vi "Listener.vi"(8 "ErrorArray":errorcluster[](array[cluster])) -> (0 "ErrorArray":errorcluster[](array[cluster]), 2 "Accepted?":bool)   [LabVIEW 2017, in "Comms.lvlib"]
uses:
  Comms.lvlib
  <userlib>/NIST/Socket Class/Classes/Socket.TCP/Socket.TCP.lvclass
  <userlib>/NIST/NISTErrorLib/NISTErrorLib.lvlib
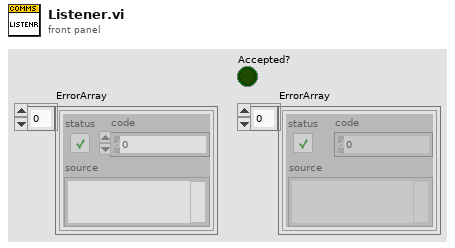
[diagram p1: front panel]
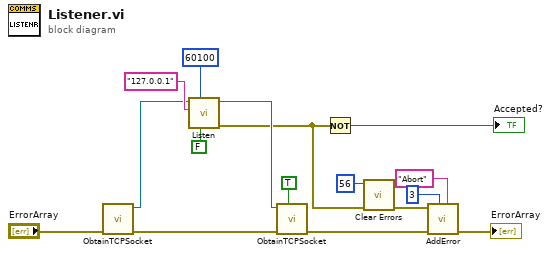
[diagram p0: block diagram]
diagram:
  n1 = call "ObtainTCPSocket.vi"("ErrorArray"="ErrorArray") -> ("ErrorArray"=w6:errorcluster[], "SocketRef"=w13:refnum<class "Socket.TCP.lvclass">)  [unwired: 9 in]
  n2 = call <userlib>:"Listen.vi"("clear_timeout_error (f)"=FALSE, "listener_port"=u16 60100, "net_address"="127.0.0.1", "Socket.TCP in"=w13) -> ("error out"=w2:errorcluster, "Socket.TCP out"=w3:refnum<class "Socket.TCP.lvclass">)  [unwired: 6 in]
  n3 = call "ObtainTCPSocket.vi"("write (f)"=TRUE, "ErrorArray"=w6, "SocketRef"=w3) -> ("ErrorArray"=w5:errorcluster[])  [unwired: 7 in, 1 out]
  n4 = Not(x=w2) -> (.not. x?=→"Accepted?":bool)
  n5 = call <vilib>:"Clear Errors.vi"("error in (no error)"=w2, "specific error code to clear (0: all)"=56) -> ("error out"=w11:errorcluster)  [unwired: 4 in, 1 out]
  n6 = call <userlib>:"AddError.vi"("Severity"="Abort", "Priority"=u8 3, "ErrorArray"=w5, "error in (no error)"=w11) -> ("ErrorArray"=→"ErrorArray":errorcluster[])  [unwired: 6 in, 1 out]
